vi "CheckIfPowerExceed.vi"(6 "Power":dbl, 7 "Role":u16, 8 "error in (no error)":errorcluster, 9 "Torque":dbl, 10 "Speed":dbl, 11 "4503 in":refnum<class "4503.lvclass">) -> (0 "error out":errorcluster, 3 "4503 out":refnum<class "4503.lvclass">)   [LabVIEW 2024, in "4503 Actor.lvlib" / "4503.lvclass"]
uses:
  4503.lvclass
  C:/Program Files (x86)/National Instruments/LabVIEW 2024/vi.lib/ActorFramework/Actor/Actor.lvclass
  <vilib>/ActorFramework/Actor/Actor.lvclass/Actor.ctl
  4503.lvclass/4503.ctl
  MFActor/ActorMessage/MF Task Name.ctl
  <vilib>/ActorFramework/Actor/Actor.lvclass
  MFActor/ActorMessage/MFActorMsg.lvclass
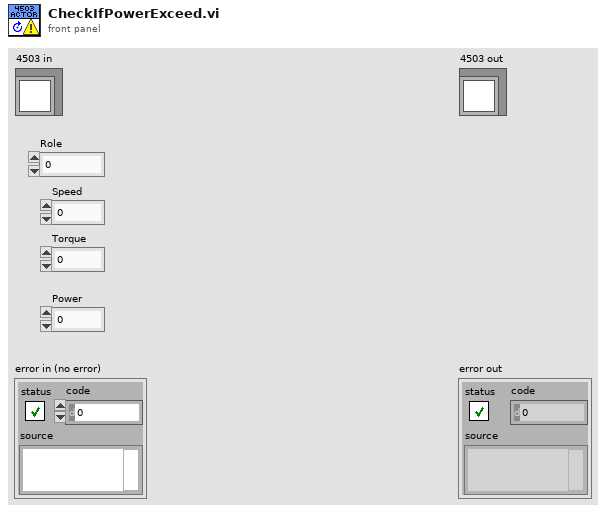
[diagram p1: front panel]
types:
  T1 = typedef "MF Task Name.ctl" = enum16{"DIChanged", "UpdateErrorCode", "SetTorque", "SetDriveTorque", "DataUpdated", "RunningTestProc", "StreamCtrl", "RunPID", "StopTest", "TCP Conn", "RefreshAutoUI", "ZeroAngle", "NestedActorLaunched", "NestedActorEnded", "ShowPsMsg"}
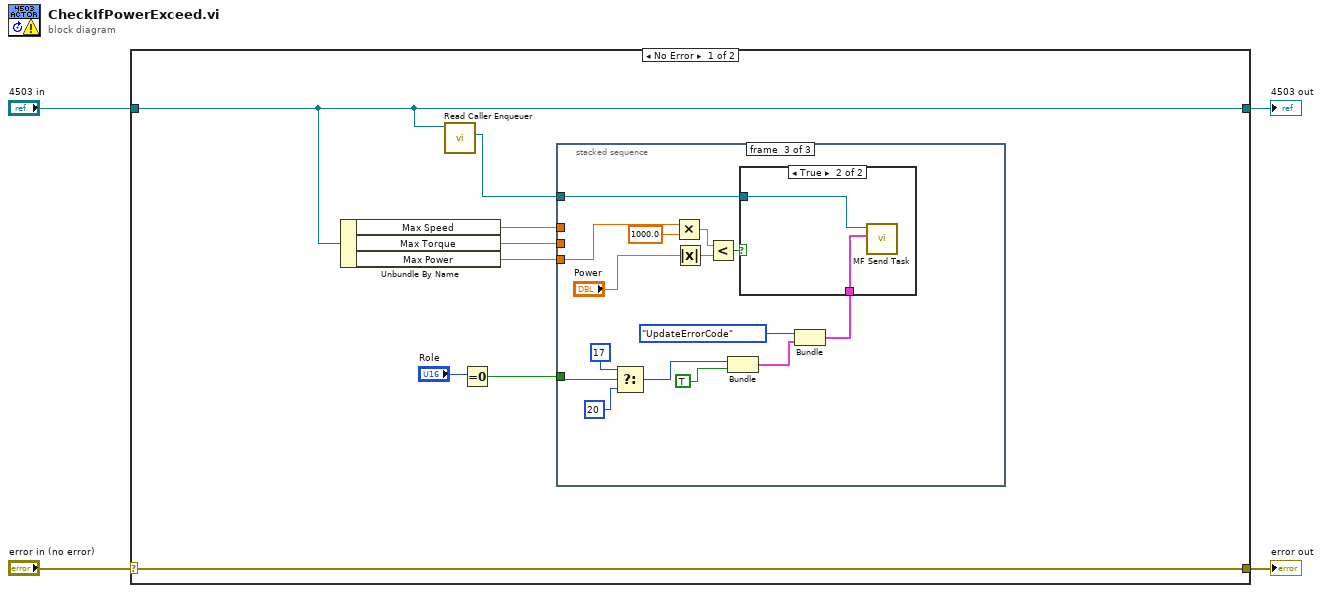
[diagram p0: block diagram]
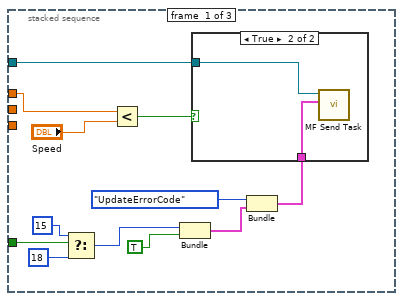
[diagram p2: hidden frame]
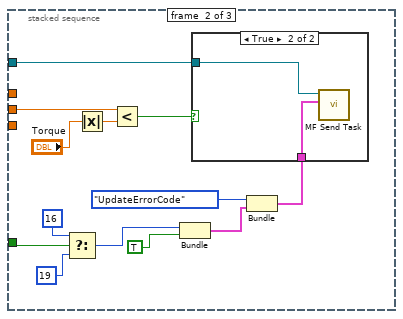
[diagram p4: hidden frame]
diagram:
  n1 = case shown="No Error" "error in (no error)" {
    selector: "error in (no error)" -> [w12 w60]
    tunnel: [w12 w60] -> w3
    tunnel: [w8 w59] -> w1
    tunnel: "4503 in" -> [w8 w59]
    frame No Error {
      n2 = Unbundle By Name(w8) -> ("Max Speed"=w11:dbl, "Max Torque"=w10:dbl, "Max Power"=w9:dbl)
      n3 = call <vilib>:"Read Caller Enqueuer.vi"("Actor"=w8) -> ("Caller Enqueuer"=w7:refnum<class "Message Enqueuer.lvclass">)  [unwired: 10 in]
      n4 = Equal To 0?(x="Role") -> (x = 0?=w5:bool)
      n5 = stacked-sequence {
        tunnel: w11 -> [w24 _ _]
        tunnel: w10 -> [_ w28 _]
        tunnel: w9 -> [_ _ w44]
        tunnel: w7 -> [w22 w39 w56]
        tunnel: w5 -> [w16 w32 w50]
        frame #0 {
          n6 = Select(t=15, s=w16, f=18) -> (s? t:f=w13:i32)
          n7 = Less?(x=w24, y="Speed") -> (x < y?=w17:bool)
          n8 = Bundle(w13, TRUE) -> (w19:cluster{i32, bool})  [unwired: 1 in]
          n9 = Bundle("MF Msg Enum"=MF_Task_Name."UpdateErrorCode", w19) -> (w18:cluster{"MF Msg Enum":T1, cluster{i32, bool}})  [unwired: 1 in]
          n10 = case shown="True" w17 {
            tunnel: w22 -> [_ w26]
            tunnel: w18 -> [_ w25]
            frame False {
            }
            frame True {
              n11 = call "MF Send Task.vi"("MsgType"=w25, "Message Enqueuer"=w26) -> ()  [unwired: 9 in, 1 out]
            }
          }
        }
        frame #1 {
          n12 = Select(t=16, s=w32, f=19) -> (s? t:f=w31:i32)
          n13 = Absolute Value(x="Torque") -> (abs(x)=w27:dbl)
          n14 = Less?(x=w28, y=w27) -> (x < y?=w34:bool)
          n15 = Bundle(w31, TRUE) -> (w36:cluster{i32, bool})  [unwired: 1 in]
          n16 = Bundle("MF Msg Enum"=MF_Task_Name."UpdateErrorCode", w36) -> (w35:cluster{"MF Msg Enum":T1, cluster{i32, bool}})  [unwired: 1 in]
          n17 = case shown="True" w34 {
            tunnel: w39 -> [_ w41]
            tunnel: w35 -> [_ w40]
            frame False {
            }
            frame True {
              n18 = call "MF Send Task.vi"("MsgType"=w40, "Message Enqueuer"=w41) -> ()  [unwired: 9 in, 1 out]
            }
          }
        }
        frame #2 {
          n19 = Select(t=17, s=w50, f=20) -> (s? t:f=w49:i32)
          n20 = Multiply(x=w44, y=1000.0) -> (x*y=w43:dbl)
          n21 = Absolute Value(x="Power") -> (abs(x)=w45:dbl)
          n22 = Less?(x=w43, y=w45) -> (x < y?=w51:bool)
          n23 = Bundle(w49, TRUE) -> (w53:cluster{i32, bool})  [unwired: 1 in]
          n24 = Bundle("MF Msg Enum"=MF_Task_Name."UpdateErrorCode", w53) -> (w52:cluster{"MF Msg Enum":T1, cluster{i32, bool}})  [unwired: 1 in]
          n25 = case shown="True" w51 {
            tunnel: w56 -> [_ w58]
            tunnel: w52 -> [_ w57]
            frame False {
            }
            frame True {
              n26 = call "MF Send Task.vi"("MsgType"=w57, "Message Enqueuer"=w58) -> ()  [unwired: 9 in, 1 out]
            }
          }
        }
      }
    }
    frame Error {
    }
  }
  "error out" <- w3
  "4503 out" <- w1
